vi "Close.vi"(8 "error in":errorcluster, 11 "CANopen Master in":refnum<class "CANopen Master.lvclass">) -> (0 "error out":errorcluster, 3 "CANopen Master out":refnum<class "CANopen Master.lvclass">)   [LabVIEW 2024, in "CANopen Master.lvclass"]
uses:
  CANopen Master.lvclass
  CANopen Master.lvclass/CANopen Master.ctl
  Example/Network Management/Network Mangement.lvclass
  SDO Manager/SDO Manager.lvclass
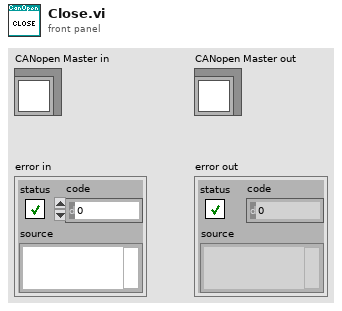
[diagram p1: front panel]
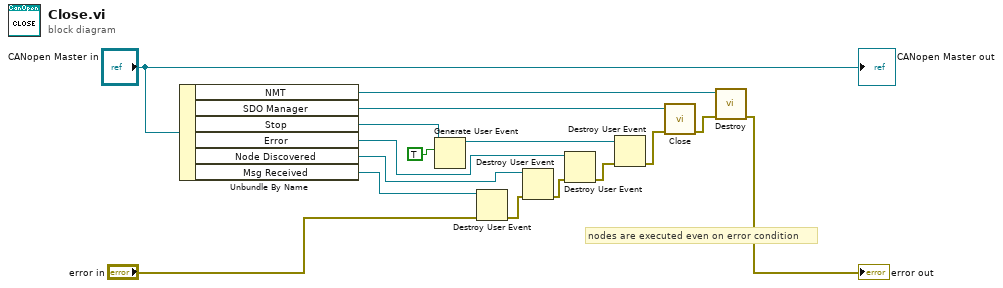
[diagram p0: block diagram]
diagram:
  # "nodes are executed even on error condition"
  n1 = Unbundle By Name("CANopen Master in") -> ("NMT"=w7:refnum<class "Network Mangement.lvclass">, "SDO Manager"=w8:refnum<class "SDO Manager.lvclass">, "Stop"=w5:refnum<user-event>, "Error"=w3:refnum<user-event>, "Node Discovered"=w2:refnum<user-event>, "Msg Received"=w1:refnum<user-event>)
  n2 = Generate User Event(user event=w5, event data cluster=TRUE ("event data")) -> (user event out=w4:refnum<user-event>)  [unwired: 2 in, 1 out]
  n3 = Destroy User Event(user event=w1, error in="error in") -> (error out=w15:errorcluster)
  n4 = Destroy User Event(user event=w2, error in=w15) -> (error out=w14:errorcluster)
  n5 = Destroy User Event(user event=w3, error in=w14) -> (error out=w16:errorcluster)
  n6 = Destroy User Event(user event=w4, error in=w16) -> (error out=w13:errorcluster)
  n7 = call "Close.vi"("Error In"=w13, "SDO Manager"=w8) -> ("Error Out"=w12:errorcluster)  [unwired: 8 in, 1 out]
  n8 = call-dynamic "Destroy.vi"("Error In"=w12, "reference in"=w7) -> ("Error Out"=→"error out":errorcluster)  [unwired: 8 in, 1 out]
  "CANopen Master out" <- "CANopen Master in"
